vi "Initialize.vi"(8 "error in (no error)":errorcluster, 9 "PPLs Folder Path":path, 10 "INI File Path":path, 11 "Device":string) -> (0 "error out":errorcluster, 3 "Digital Delay Generator out":refnum<class "Digital Delay Generator.lvclass">)   [LabVIEW 2018, in "Digital Delay Generator.lvlib" / "Digital Delay Generator.lvclass"]
uses:
  Digital Delay Generator.lvclass
  Digital Delay Generator.lvclass/Digital Delay Generator.ctl
  PPLs/Configuration/Configuration.lvlibp/Configuration.lvclass
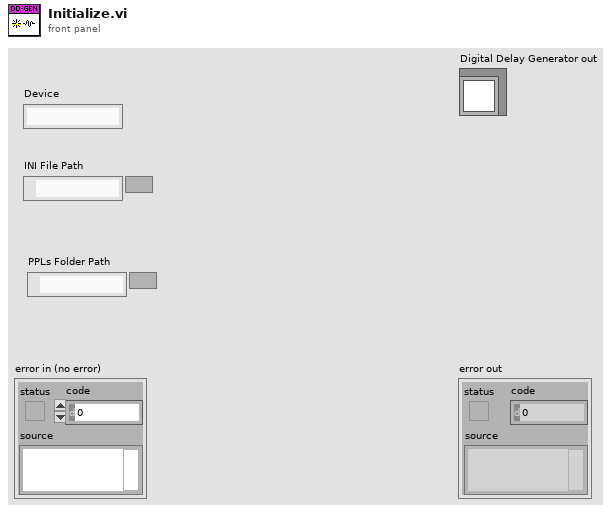
[diagram p1: front panel]
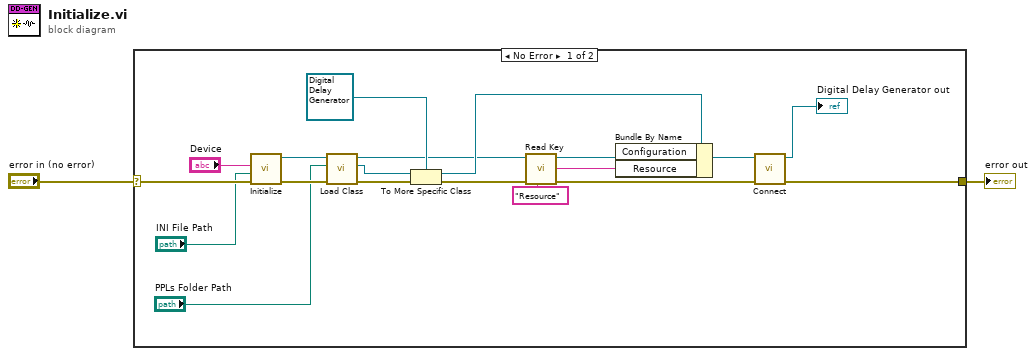
[diagram p0: block diagram]
diagram:
  n1 = case shown="No Error" "error in (no error)" {
    selector: "error in (no error)" -> [w21 w22]
    tunnel: [w6 w22] -> w1
    frame No Error {
      n2 = call "Initialize.vi"("error in"=w21, "INI File Path"="INI File Path", "Device"="Device") -> ("error out"=w19:errorcluster, "Configuration out"=w18:refnum<class "Configuration.lvclass">)  [unwired: 7 in]
      n3 = call "Load Class.vi"("error in"=w19, "PPLs Folder Path"="PPLs Folder Path", "Configuration in"=w18) -> ("error out"=w17:errorcluster, "Class out"=w16:refnum<class>, "Configuration out"=w13:refnum<class "Configuration.lvclass">)  [unwired: 6 in]
      n4 = To More Specific Class(target class=refnum<class "Digital Delay Generator.lvclass"> refnum ("Digital Delay Generator in"), reference=w16, error in=w17) -> (specific class reference=w14:refnum<class "Digital Delay Generator.lvclass">, error out=w11:errorcluster)
      n5 = call "Read Key.vi"("Key:"="Resource", "error in"=w11, "Configuration in"=w13) -> ("error out"=w8:errorcluster, "Value"=w9:string, "Configuration out"=w12:refnum<class "Configuration.lvclass">)  [unwired: 6 in]
      n6 = Bundle By Name(cluster=w14, "Configuration"=w12, "Resource"=w9) -> (w7:refnum<class "Digital Delay Generator.lvclass">)
      n7 = call-dynamic "Connect.vi"("error in (no error)"=w8, "Digital Delay Generator in"=w7) -> ("error out"=w6:errorcluster, "Digital Delay Generator out"=→"Digital Delay Generator out":refnum<class "Digital Delay Generator.lvclass">)  [unwired: 8 in]
    }
    frame Error {
    }
  }
  "error out" <- w1
